vi "RC_PWM_to_01.vi"(8 "error in (no error)":errorcluster, 11 "Refnum in":refnum<k20>) -> (0 "error out":errorcluster, 1 "Sail Control Output":dbl, 2 "Rudder Control Output":dbl, 3 "Hand Sail Control":T1 {"MainSailSuggestion" min=0.0 max=1.0; "JibSailSuggestion" min=0.0 max=1.0})   [LabVIEW 2013]
doc: "This VI takes the PWM read FPGA code and reads values from the controller. We determined via testing the constants that let us take PWM values and convert them to 0,1 for the sails and -1,1 for the sails.\n\nThere is jitter detection in this code. If the command value changed by less than 0.03 from the last command, then the command is unchanged from before. This removes a constant small jitter from the read PWM value.\n\nEric Schneider, December 2014"
uses:
  Data/TypeDefs/Sail Set Suggestions.ctl
  <vilib>/rvi/interface/common/niFpgaWaitOnOcc.vi
  <vilib>/Utility/error.llb/Error Cluster From Error Code.vi
  <vilib>/rvi/errors/niLvFpgaAdjustHostInterfaceError.vi
  <vilib>/rvi/interface/nirviReadWriteControl/nirviReadWriteControl.xnode
  NiFpgaLv.dll
  <vilib>/rvi/interface/Simulation/niFpgaSimulationCallBeginRW.vi
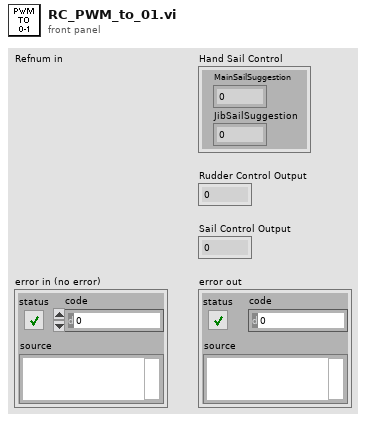
[diagram p1: front panel]
types:
  T1 = typedef "Sail Set Suggestions.ctl" = cluster{"MainSailSuggestion":dbl, "JibSailSuggestion":dbl}
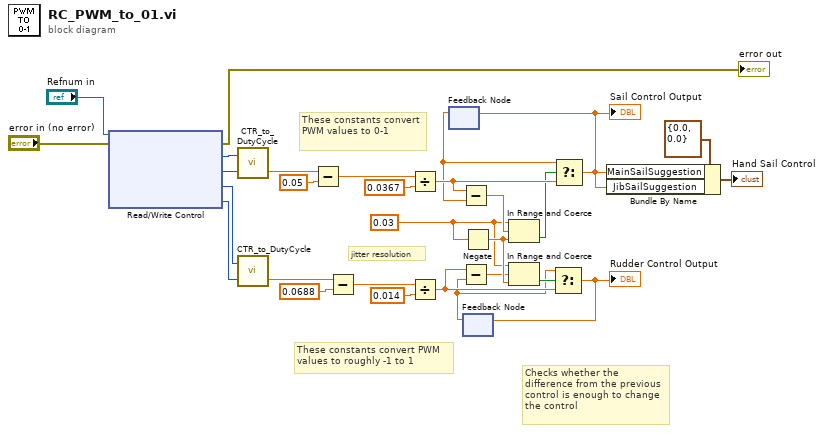
[diagram p0: block diagram]
diagram:
  w1 = 0.03 ("Jitter cutout")
  # "These constants convert PWM values to roughly -1 to 1"
  # "These constants convert PWM values to 0-1"
  # "Checks whether the difference from the previous control is enough to change the control"
  # "jitter resolution"
  n1 = xnode "Read/Write Control"("FPGA VI Reference In"="Refnum in", "error in"="error in (no error)") -> ("error out"=→"error out":errorcluster, "Sail High Center"=w10:u32, "Sail Low Center"=w11:u32, "Rudder High Center"=w12:u32, "Rudder Low Center"=w13:u32)  [unwired: 1 out]
  n2 = call "CTR_to_DutyCycle.vi"("LOW CTR"=w11, "HIGH CTR"=w10) -> ("duty cycle fraction [0-1]"=w15:dbl)  [unwired: 1 out]
  n3 = call "CTR_to_DutyCycle.vi"("LOW CTR"=w13, "HIGH CTR"=w12) -> ("duty cycle fraction [0-1]"=w21:dbl)  [unwired: 1 out]
  n4 = Subtract(x=w15, y=0.05) -> (x-y=w16:dbl)
  n5 = Subtract(x=w21, y=0.0688) -> (x-y=w19:dbl)
  n6 = Divide(x=w16, y=0.0367) -> (x/y=w29:dbl)
  n7 = Divide(x=w19, y=0.014) -> (x/y=w26:dbl)
  n8 = feedback #1() -> (w7:dbl)  [unwired: 1 in]
  n9 = Subtract(x=w29, y=w7) -> (x-y=w22:dbl)
  n10 = Negate(x=w1) -> (-x=w28:dbl)
  n11 = feedback #2() -> (w9:dbl)  [unwired: 1 in]
  n12 = Subtract(x=w26, y=w9) -> (x-y=w24:dbl)
  n13 = In Range and Coerce(upper limit=w1, x=w22, lower limit=w28) -> (In Range?=w23:bool)  [unwired: 1 out]
  n14 = In Range and Coerce(upper limit=w1, x=w24, lower limit=w28) -> (In Range?=w25:bool)  [unwired: 1 out]
  n15 = Select(t=w9, s=w25, f=w26) -> (s? t:f=w8:dbl)
  "Rudder Control Output" <- w8
  n16 = feedback-in #2(w8) -> ()
  n17 = Select(t=w7, s=w23, f=w29) -> (s? t:f=w6:dbl)
  "Sail Control Output" <- w6
  n18 = feedback-in #1(w6) -> ()
  n19 = Bundle By Name(cluster=T1 {"MainSailSuggestion"=0.0, "JibSailSuggestion"=0.0} ("Hand Sail Control"), "MainSailSuggestion"=w6, "JibSailSuggestion"=w6) -> (→"Hand Sail Control":T1)
